vi "Write_1D_Array.vi"(6 "Array To Write":dbl[][](array[numeric])=[[0.0]], 8 "error in (no error)":errorcluster, 9 "Cell Range 2":string="B2", 10 "Cell Range 1":string="A2", 11 "Automation Refnum in":refnum<k7>) -> (0 "error out":errorcluster, 3 "Automation Refnum out":refnum<k7>)   [LabVIEW 2014]
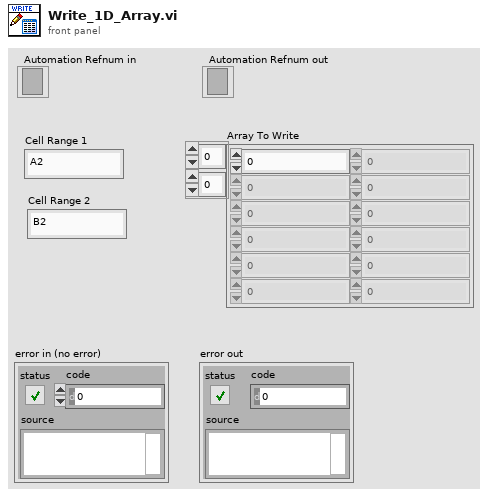
[diagram p1: front panel]
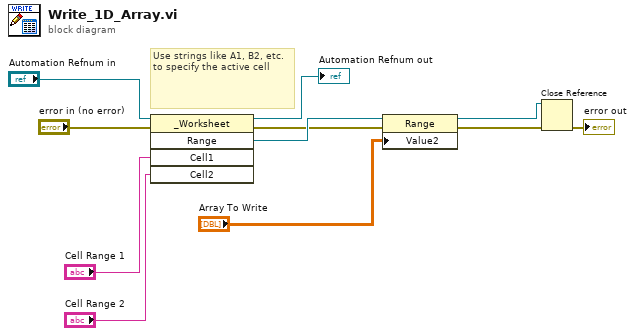
[diagram p0: block diagram]
diagram:
  # "Use strings like A1, B2, etc. to specify the active cell"
  n1 = invoke class="_Worksheet" method="Range"(reference="Automation Refnum in", error in="error in (no error)", "Cell1"="Cell Range 1", "Cell2"="Cell Range 2") -> (reference out=→"Automation Refnum out":refnum<k7>, error out=w2:errorcluster, "Range"=w3:refnum<k7>)  [unwired: 1 in, 2 out]
  n2 = property class="Range"(reference=w3, error in=w2, "Value2"="Array To Write") -> (reference out=w9:refnum<k7>, error out=w10:errorcluster)
  n3 = Close Reference(reference=w9, error in (no error)=w10) -> (error out=→"error out":errorcluster)
